vi "Configure Acquisition.vi"(0 "VISA resource name":refnum<visa-resource-name>, 1 "Auto Scaling (T: Enable)":bool=TRUE, 2 "Vertical Scale (0: Logarithmic)":i32(ring) items=["Logarithmic", "Linear"], 3 "Trace Name (1: Trace 1)":i32(ring)=1 items=["Trace 1"=1, "Trace 2"=2, "Trace 3"=3, "Trace 4"=4, "Trace 5"=5, "Trace 6"=6], 5 "Enable Continuous Sweep (T: Enable)":bool=TRUE, 7 "Auto Detector (T: Enable)":bool=TRUE, 9 "Manual Detector Type (0: Normal)":i32(ring) items=["Normal", "Average", "Peak", "Sample", "Negative peak"], 11 "error in (no error)":errorcluster, 12 "Scale Per Division (10 dB)":dbl=10.0, 13 "Sweep Points (1001)":i32=1001) -> (4 "VISA resource name out":refnum<visa-resource-name>, 15 "error out":errorcluster)   [LabVIEW 2014, in "Agilent MXA Series.lvlib"]
doc: "Configures the acquisition properties of the spectrum analyzer."
uses:
  Agilent MXA Series.lvlib
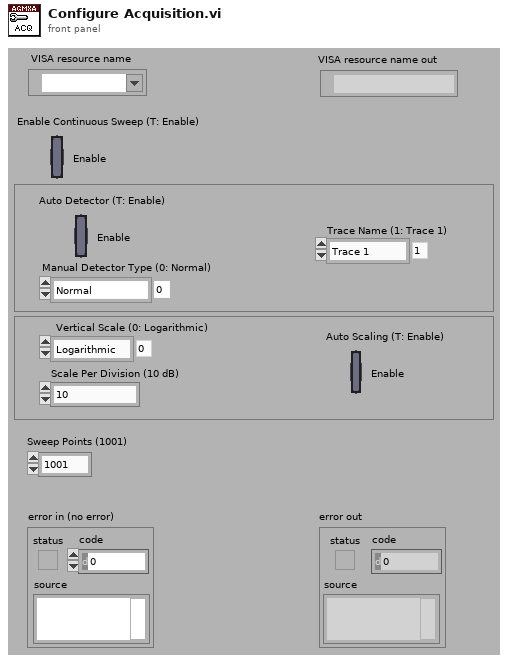
[diagram p1: front panel]
types:
  T1 = typedef "Agilent MXA Series.lvlib/Extended User Data.ctl" = cluster{"Measurement Type":i32, "Agilent MXA/EXA Model":i32}
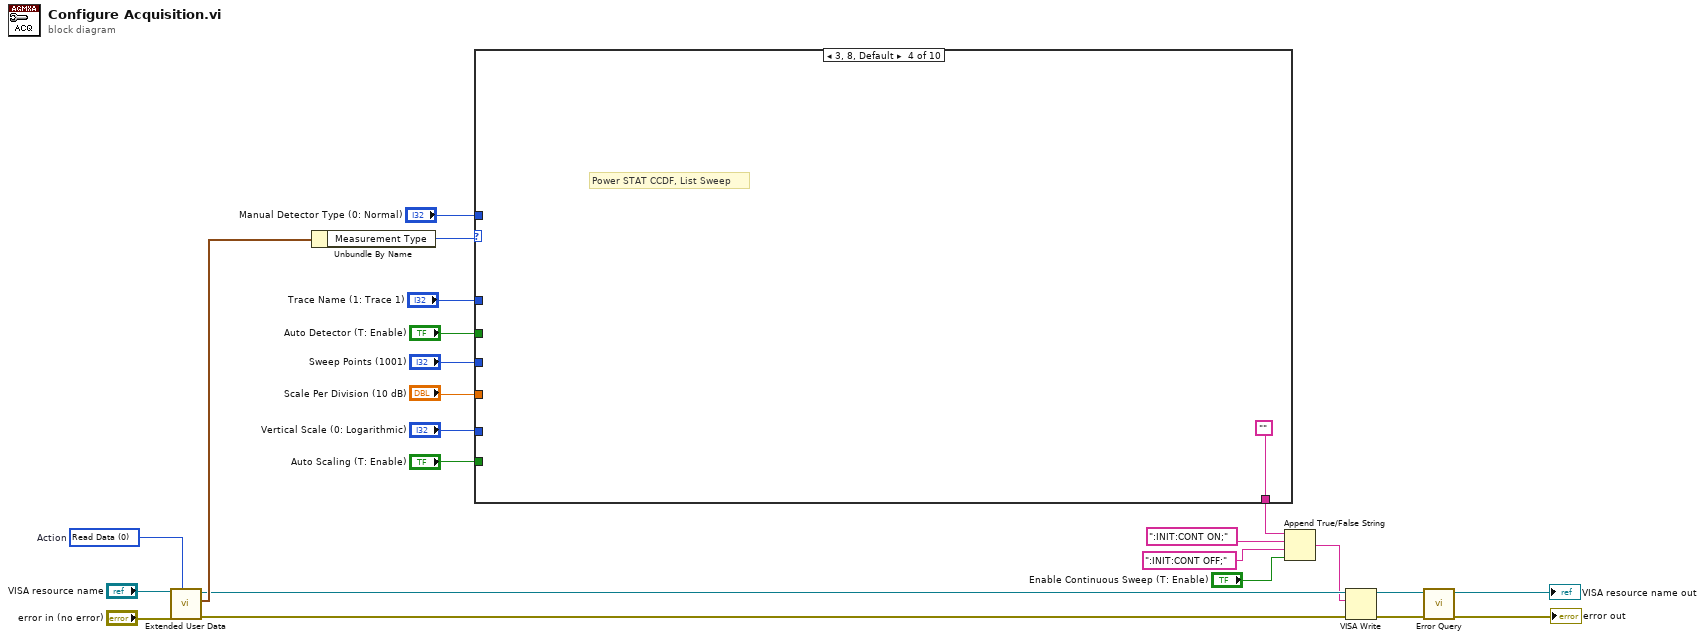
[diagram p0: block diagram]
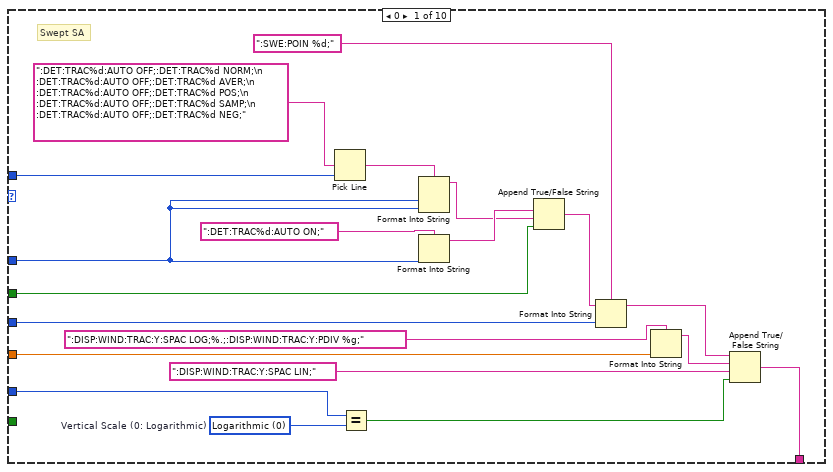
[diagram p2: hidden frame]
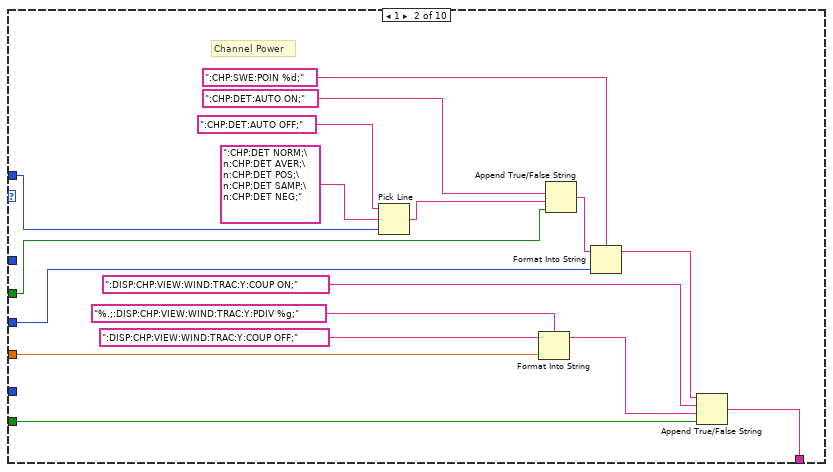
[diagram p3: hidden frame]
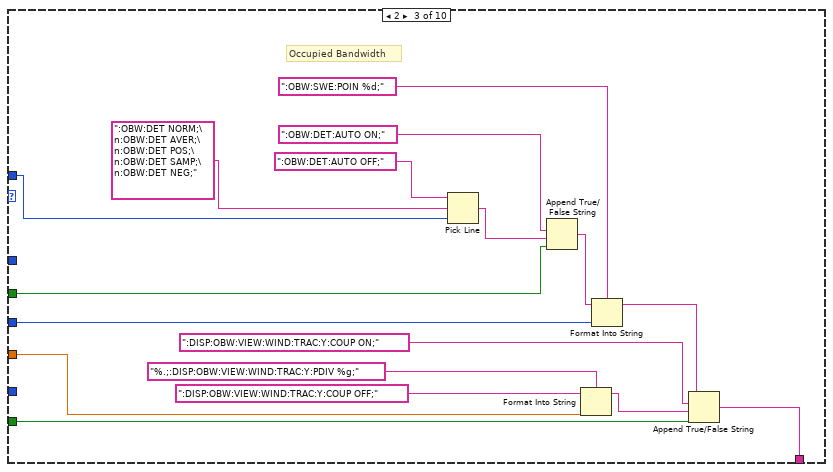
[diagram p4: hidden frame]
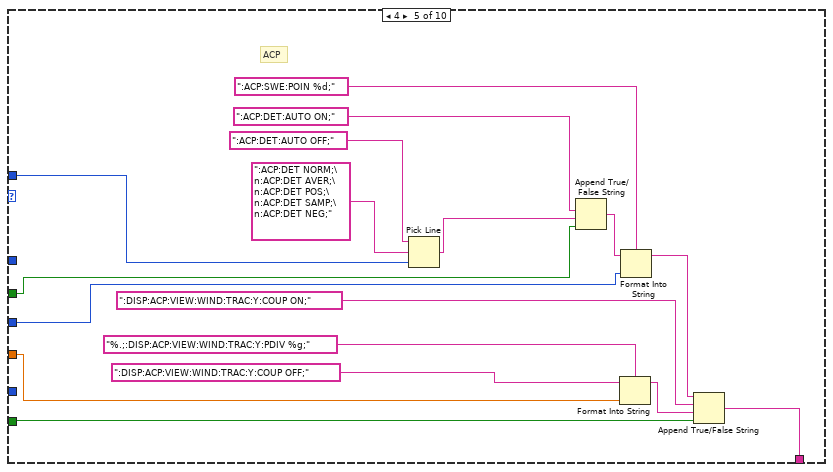
[diagram p5: hidden frame]
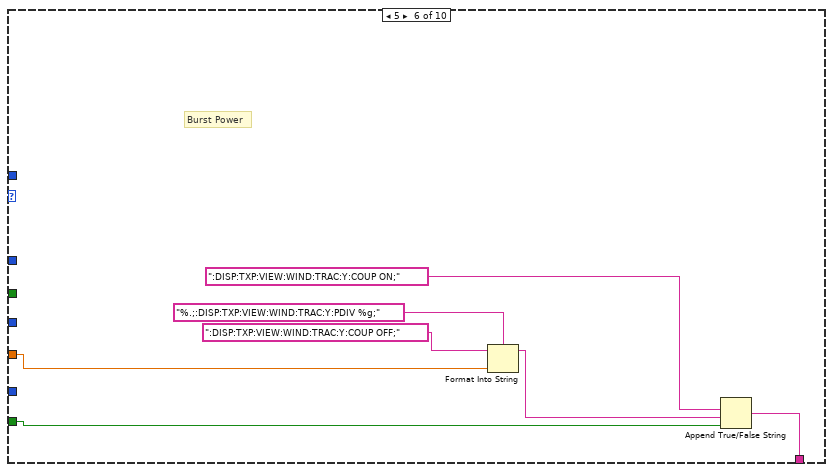
[diagram p6: hidden frame]
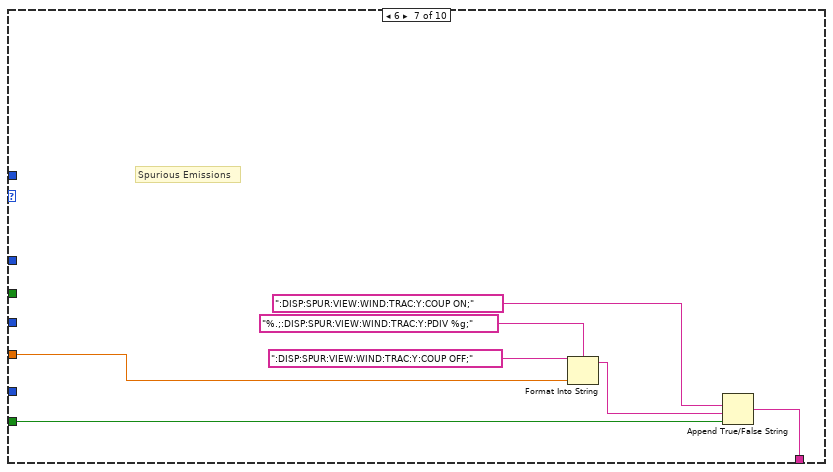
[diagram p7: hidden frame]
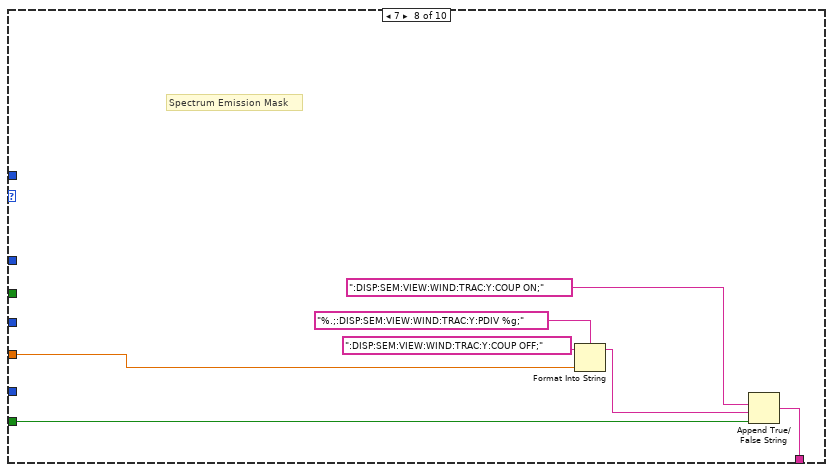
[diagram p8: hidden frame]
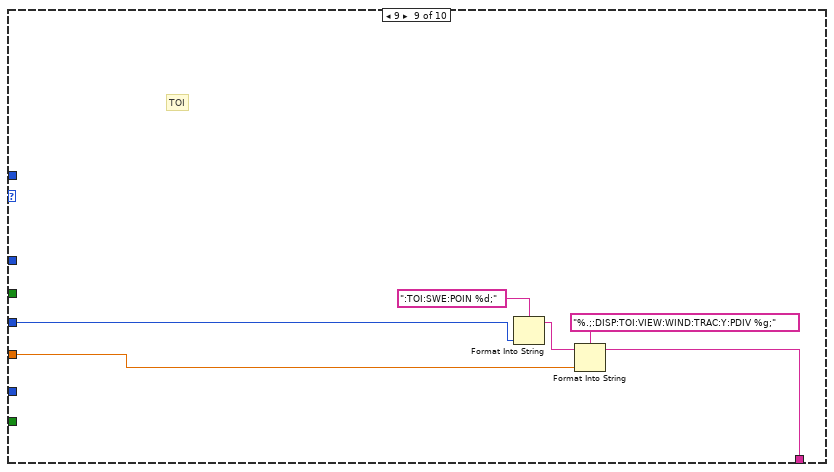
[diagram p9: hidden frame]
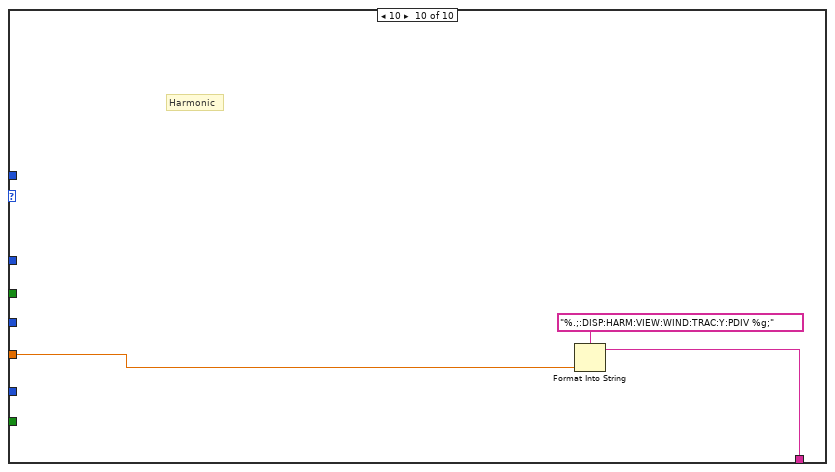
[diagram p10: hidden frame]
diagram:
  w1 = 0 items=["Read Data", "Write Data", "Clear Data", "Clear ALL Data"]  # Action
  n1 = call "Extended User Data.vi"("Action (1:Write Data)"=w1, "Error In (no error)"="error in (no error)", "VISA resource name in"="VISA resource name") -> ("Error Out"=w7:errorcluster, "User Data Out"=w21:T1, "VISA resource name out"=w8:refnum<visa-resource-name>)  [unwired: 6 in]
  n2 = Unbundle By Name(w21) -> ("Measurement Type"=w20:i32)
  n3 = case shown="3, 8, Default" w20 {
    tunnel: "Manual Detector Type (0: Normal)" -> [w25 w57 w71 _ w87 _ _ _ _ _]
    tunnel: "Trace Name (1: Trace 1)" -> [w24 _ _ _ _ _ _ _ _ _]
    tunnel: "Auto Detector (T: Enable)" -> [w31 w56 w70 _ w86 _ _ _ _ _]
    tunnel: "Sweep Points (1001)" -> [w41 w54 w69 _ w85 _ _ _ w117 _]
    tunnel: "Scale Per Division (10 dB)" -> [w38 w51 w67 _ w84 w100 w105 w114 w121 w124]
    tunnel: "Vertical Scale (0: Logarithmic)" -> [w35 _ _ _ _ _ _ _ _ _]
    tunnel: "Auto Scaling (T: Enable)" -> [_ w50 w66 _ w83 w99 w107 w113 _ _]
    tunnel: [w37 w48 w65 "" ("output string") w82 w98 w106 w112 w120 w123] -> w10
    frame 0 {
      w34 = 0 items=["Logarithmic", "Linear"]  # Vertical Scale (0: Logarithmic)
      # "Swept SA"
      n4 = Pick Line(multi-line string=":DET:TRAC%d:AUTO OFF;:DET:TRAC%d NORM;\n :DET:TRAC%d:AUTO OFF;:DET:TRAC%d AVER;\n :DET:TRAC%d:AUTO OFF;:DET:TRAC%d POS;\n :DET:TRAC%d:AUTO OFF;:DET:TRAC%d SAMP;\n :DET:TRAC%d:AUTO OFF;:DET:TRAC%d NEG;", line index=w25) -> (output string=w32:string)  [unwired: 1 in]
      n5 = Equal?(x=w35, y=w34) -> (x = y?=w33:bool)
      n6 = Format Into String(format string=w32, w24, w24) -> (resulting string=w29:string)  [unwired: 2 in, 1 out]
      n7 = Format Into String(format string=":DET:TRAC%d:AUTO ON;", w24) -> (resulting string=w30:string)  [unwired: 2 in, 1 out]
      n8 = Append True/False String(1:w31, 2:w29, 3:w30) -> (0:w40:string)  [unwired: 1 in]
      n9 = Format Into String(format string=":SWE:POIN %d;", initial string=w40, w41) -> (resulting string=w28:string)  [unwired: 1 in, 1 out]
      n10 = Format Into String(format string=":DISP:WIND:TRAC:Y:SPAC LOG;%.;:DISP:WIND:TRAC:Y:PDIV %g;", w38) -> (resulting string=w27:string)  [unwired: 2 in, 1 out]
      n11 = Append True/False String(1:w33, 2:":DISP:WIND:TRAC:Y:SPAC LIN;" ("string (\"\")"), 3:w27, 4:w28) -> (0:w37:string)
    }
    frame 1 {
      # "Channel Power"
      n12 = Pick Line(string ("")=":CHP:DET:AUTO OFF;" ("string"), multi-line string=":CHP:DET NORM;\n:CHP:DET AVER;\n:CHP:DET POS;\n:CHP:DET SAMP;\n:CHP:DET NEG;", line index=w57) -> (output string=w55:string)
      n13 = Format Into String(format string="%.;:DISP:CHP:VIEW:WIND:TRAC:Y:PDIV %g;", initial string=":DISP:CHP:VIEW:WIND:TRAC:Y:COUP OFF;" ("true string"), w51) -> (resulting string=w44:string)  [unwired: 1 in, 1 out]
      n14 = Append True/False String(1:w56, 2:w55, 3:":CHP:DET:AUTO ON;" ("string")) -> (0:w52:string)  [unwired: 1 in]
      n15 = Format Into String(format string=":CHP:SWE:POIN %d;", initial string=w52, w54) -> (resulting string=w45:string)  [unwired: 1 in, 1 out]
      n16 = Append True/False String(1:w50, 2:w44, 3:":DISP:CHP:VIEW:WIND:TRAC:Y:COUP ON;" ("true string"), 4:w45) -> (0:w48:string)
    }
    frame 2 {
      # "Occupied Bandwidth"
      n17 = Pick Line(string ("")=":OBW:DET:AUTO OFF;" ("string"), multi-line string=":OBW:DET NORM;\n:OBW:DET AVER;\n:OBW:DET POS;\n:OBW:DET SAMP;\n:OBW:DET NEG;", line index=w71) -> (output string=w74:string)
      n18 = Append True/False String(1:w70, 2:w74, 3:":OBW:DET:AUTO ON;" ("string")) -> (0:w72:string)  [unwired: 1 in]
      n19 = Format Into String(format string="%.;:DISP:OBW:VIEW:WIND:TRAC:Y:PDIV %g;", initial string=":DISP:OBW:VIEW:WIND:TRAC:Y:COUP OFF;" ("true string"), w67) -> (resulting string=w61:string)  [unwired: 1 in, 1 out]
      n20 = Format Into String(format string=":OBW:SWE:POIN %d;", initial string=w72, w69) -> (resulting string=w62:string)  [unwired: 1 in, 1 out]
      n21 = Append True/False String(1:w66, 2:w61, 3:":DISP:OBW:VIEW:WIND:TRAC:Y:COUP ON;" ("true string"), 4:w62) -> (0:w65:string)
    }
    frame 3, 8, Default {
      # "Power STAT CCDF, List Sweep"
    }
    frame 4 {
      # "ACP"
      n22 = Pick Line(string ("")=":ACP:DET:AUTO OFF;" ("string"), multi-line string=":ACP:DET NORM;\n:ACP:DET AVER;\n:ACP:DET POS;\n:ACP:DET SAMP;\n:ACP:DET NEG;", line index=w87) -> (output string=w92:string)
      n23 = Append True/False String(1:w86, 2:w92, 3:":ACP:DET:AUTO ON;" ("string")) -> (0:w90:string)  [unwired: 1 in]
      n24 = Format Into String(format string="%.;:DISP:ACP:VIEW:WIND:TRAC:Y:PDIV %g;", initial string=":DISP:ACP:VIEW:WIND:TRAC:Y:COUP OFF;" ("true string"), w84) -> (resulting string=w79:string)  [unwired: 1 in, 1 out]
      n25 = Format Into String(format string=":ACP:SWE:POIN %d;", initial string=w90, w85) -> (resulting string=w80:string)  [unwired: 1 in, 1 out]
      n26 = Append True/False String(1:w83, 2:w79, 3:":DISP:ACP:VIEW:WIND:TRAC:Y:COUP ON;" ("true string"), 4:w80) -> (0:w82:string)
    }
    frame 5 {
      # "Burst Power"
      n27 = Format Into String(format string="%.;:DISP:TXP:VIEW:WIND:TRAC:Y:PDIV %g;", initial string=":DISP:TXP:VIEW:WIND:TRAC:Y:COUP OFF;" ("true string"), w100) -> (resulting string=w96:string)  [unwired: 1 in, 1 out]
      n28 = Append True/False String(1:w99, 2:w96, 3:":DISP:TXP:VIEW:WIND:TRAC:Y:COUP ON;" ("true string")) -> (0:w98:string)  [unwired: 1 in]
    }
    frame 6 {
      # "Spurious Emissions"
      n29 = Format Into String(format string="%.;:DISP:SPUR:VIEW:WIND:TRAC:Y:PDIV %g;", initial string=":DISP:SPUR:VIEW:WIND:TRAC:Y:COUP OFF;" ("true string"), w105) -> (resulting string=w103:string)  [unwired: 1 in, 1 out]
      n30 = Append True/False String(1:w107, 2:w103, 3:":DISP:SPUR:VIEW:WIND:TRAC:Y:COUP ON;" ("true string")) -> (0:w106:string)  [unwired: 1 in]
    }
    frame 7 {
      # "Spectrum Emission Mask"
      n31 = Format Into String(format string="%.;:DISP:SEM:VIEW:WIND:TRAC:Y:PDIV %g;", initial string=":DISP:SEM:VIEW:WIND:TRAC:Y:COUP OFF;" ("true string"), w114) -> (resulting string=w110:string)  [unwired: 1 in, 1 out]
      n32 = Append True/False String(1:w113, 2:w110, 3:":DISP:SEM:VIEW:WIND:TRAC:Y:COUP ON;" ("true string")) -> (0:w112:string)  [unwired: 1 in]
    }
    frame 9 {
      # "TOI"
      n33 = Format Into String(format string=":TOI:SWE:POIN %d;", w117) -> (resulting string=w119:string)  [unwired: 2 in, 1 out]
      n34 = Format Into String(format string="%.;:DISP:TOI:VIEW:WIND:TRAC:Y:PDIV %g;", initial string=w119, w121) -> (resulting string=w120:string)  [unwired: 1 in, 1 out]
    }
    frame 10 {
      # "Harmonic"
      n35 = Format Into String(format string="%.;:DISP:HARM:VIEW:WIND:TRAC:Y:PDIV %g;", w124) -> (resulting string=w123:string)  [unwired: 2 in, 1 out]
    }
  }
  n36 = Append True/False String(1:"Enable Continuous Sweep (T: Enable)", 2:":INIT:CONT OFF;" ("false string"), 3:":INIT:CONT ON;" ("format string"), 4:w10) -> (0:w6:string)
  n37 = VISA Write(VISA resource name=w8, write buffer=w6, error in (no error)=w7) -> (VISA resource name out=w5:refnum<visa-resource-name>, error out=w4:errorcluster)  [unwired: 1 out]
  n38 = call "Error Query.vi"("error in (no error)"=w4, "VISA resource name"=w5) -> ("error out"=→"error out":errorcluster, "VISA resource name out"=→"VISA resource name out":refnum<visa-resource-name>)  [unwired: 6 in, 2 out]
